vi "UTIL_Get5ptCalCoef.vi"() -> ()   [LabVIEW 2024]
uses:
  <vilib>/Analysis/NI_AALPro.lvlib
panel:
  out "B":dbl
  out "M":dbl
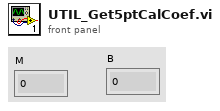
[diagram p1: front panel]
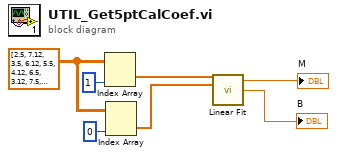
[diagram p0: block diagram]
diagram:
  w5 = dbl[][] [[2.5, 7.12], [3.5, 6.12], [5.5, 4.12], [6.5, 3.12], [7.5, 2.12]] ("Calibraion  default")
  n1 = Index Array(array=w5, index (col)=1 ("disabled index (col)")) -> (element=w4:dbl[])  [unwired: 1 in]
  n2 = Index Array(array=w5, index (col)=0 ("disabled index (col)")) -> (element=w3:dbl[])  [unwired: 1 in]
  n3 = call <vilib>:"Linear Fit.vi"("Y"=w4, "X"=w3) -> ("slope"=→"M":dbl, "intercept"=→"B":dbl)  [unwired: 9 in, 3 out]
